vi "Scale Channel.vi"(8 "error in (no error)":errorcluster, 9 "Instance":string, 10 "Value In":dbl, 11 "Lookup Table in":refnum<class "Lookup Table.lvclass">) -> (0 "error out":errorcluster, 2 "Value Out":dbl, 3 "Lookup Table out":refnum<class "Lookup Table.lvclass">)   [LabVIEW 2018, in "Lookup Table.lvclass"]
doc: "Lookup Table.lvclass:Scale Channel.vi\n\nThis VI scales a single Channel using a Lookup Table scaling.\n\nInstrument Communication Module Version 1.0\nNovember, 2017 Original Code Consulting David Thomson\n www.originalcode.com David Thomson"
uses:
  Lookup Table.lvclass
  Lookup Table.lvclass/Lookup Table.ctl
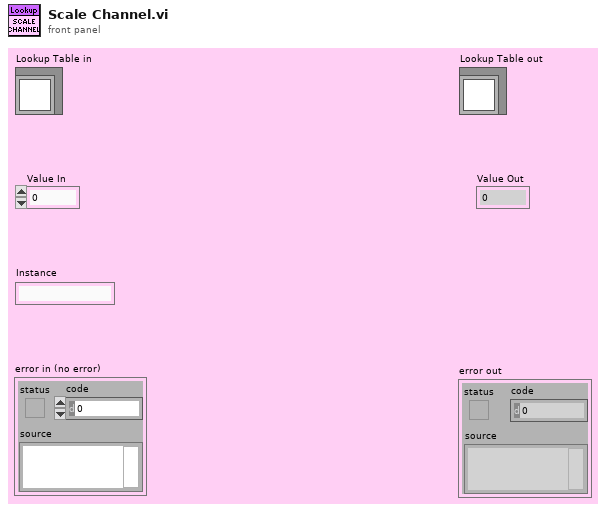
[diagram p1: front panel]
types:
  T1 = cluster{"Instance":string, "Table":cluster{"Raw Value":dbl, "Sca;ed Value":dbl}[]}[]
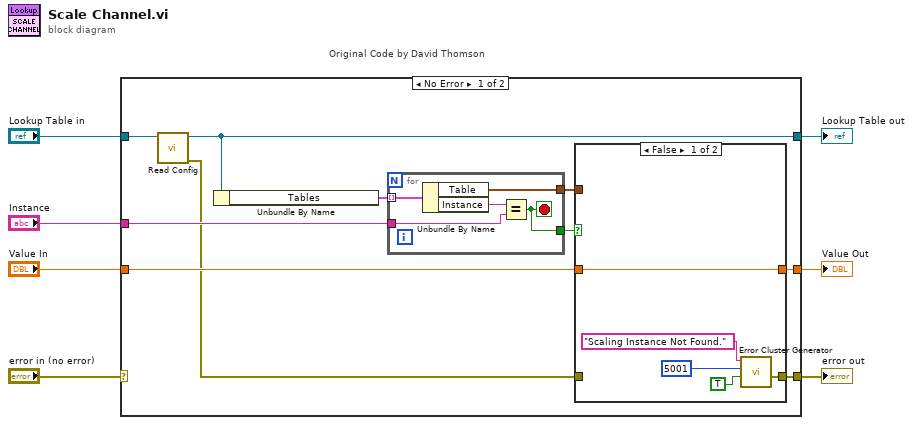
[diagram p0: block diagram]
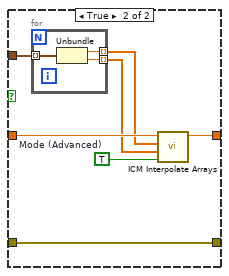
[diagram p2: hidden frame]
diagram:
  n1 = case "Original Code by David Thomson" shown="No Error" "error in (no error)" {
    selector: "error in (no error)" -> [_ w40]
    tunnel: [w14 w40] -> w6
    tunnel: [w9 w39] -> w4
    tunnel: "Lookup Table in" -> [w10 w39]
    tunnel: "Instance" -> [w17 _]
    tunnel: "Value In" -> [w12 w38]
    tunnel: [w13 w38] -> w1
    frame No Error {
      n2 = call-dynamic "Read Config.vi"("Lookup Table in"=w10) -> ("error out"=w8:errorcluster, "Lookup Table out"=w9:refnum<class "Lookup Table.lvclass">)  [unwired: 9 in]
      n3 = Unbundle By Name(w9) -> ("Tables"=w16:T1)
      n4 = for {
        tunnel: w17 -> [w35]
        tunnel: w16 -> [w37] mode=indexing
        tunnel: [w34] -> w15
        tunnel: [w33] -> w11
        stop <- w34 stop-if-true
        n5 = Unbundle By Name(w37) -> ("Table"=w33:cluster{"Raw Value":dbl, "Sca;ed Value":dbl}[], "Instance"=w36:string)
        n6 = Equal?(x=w36, y=w35) -> (x = y?=w34:bool)
      }
      n7 = case shown="False" w15 {
        tunnel: w8 -> [_ w29]
        tunnel: [w21 w29] -> w14
        tunnel: [w22 w27] -> w13
        tunnel: w12 -> [w22 w28]
        tunnel: w11 -> [_ w26]
        frame False {
          n8 = call "Error Cluster Generator.vi"("Error (T)"=TRUE, "code"=5001, "Additional message"="Scaling Instance Not Found.") -> ("error out"=w21:errorcluster)  [unwired: 3 in, 1 out]
        }
        frame True {
          w23 = TRUE  # Mode (Advanced)
          n9 = for {
            tunnel: w26 -> [w32] mode=indexing
            tunnel: [w31] -> w25 mode=indexing
            tunnel: [w30] -> w24 mode=indexing
            n10 = Unbundle(w32) -> ("Raw Value"=w31:dbl, "Sca;ed Value"=w30:dbl)
          }
          n11 = call "ICM Interpolate Arrays.vi"("Mode (Advanced)"=w23, "Scaled Array"=w24, "Raw Array"=w25, "Data In"=w28) -> ("Data Out"=w27:dbl)  [unwired: 7 in]
        }
      }
    }
    frame Error {
    }
  }
  "error out" <- w6
  "Lookup Table out" <- w4
  "Value Out" <- w1
